vi "SineWaver.vi"() -> ()   [LabVIEW 2014, in "examples.lvlib"]
uses:
  examples.lvlib
  sinewavercontrols.vi
panel:
  out "Sine":dynamicdata(graph)
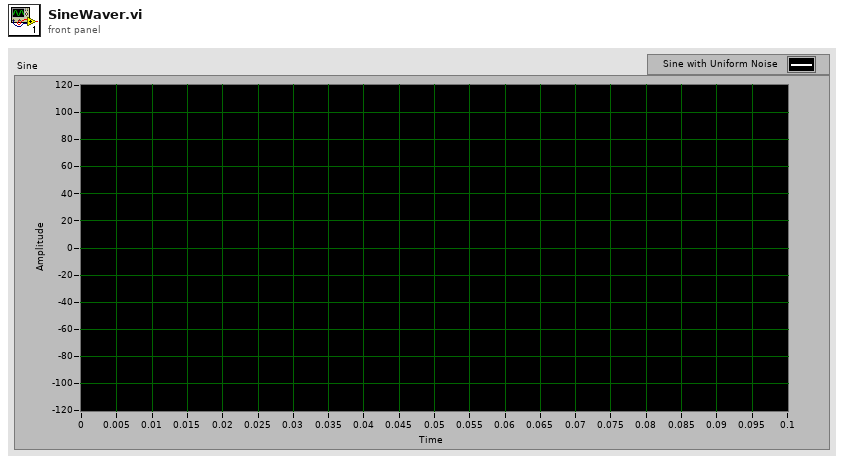
[diagram p1: front panel]
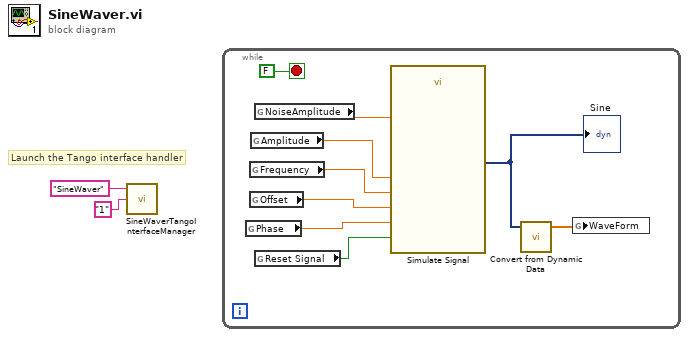
[diagram p0: block diagram]
diagram:
  # "Launch the Tango interface handler"
  n1 = call "SineWaverTangoInterfaceManager.vi"("Instance Name"="1", "Executable Name"="SineWaver") -> ()  [unwired: 1 in]
  n2 = while {
    stop <- FALSE stop-if-true
    n3 = global read "sinewavercontrols.vi" "Phase"() -> (w10:dbl)
    n4 = global read "sinewavercontrols.vi" "Frequency"() -> (w7:dbl)
    n5 = global read "sinewavercontrols.vi" "Offset"() -> (w11:dbl)
    n6 = global read "sinewavercontrols.vi" "Amplitude"() -> (w6:dbl)
    n7 = global read "sinewavercontrols.vi" "NoiseAmplitude"() -> (w8:dbl)
    n8 = global read "sinewavercontrols.vi" "Reset Signal"() -> (w3:bool)
    n9 = call "Simulate Signal"("Offset"=w11, "Reset Signal"=w3, "Frequency"=w7, "Amplitude"=w6, "Phase"=w10, "Noise amplitude"=w8) -> ("Sine with Uniform Noise"=w5:dynamicdata)  [unwired: 8 in, 1 out]
    "Sine" <- w5
    n10 = call "Convert from Dynamic Data"("Dynamic Data Type"=w5) -> ("Array"=w4:dbl[])  [unwired: 3 in]
    n11 = global write "sinewavercontrols.vi" "WaveForm"(w4) -> ()
  }
